vi "Split string by delimiter.vi"(7 "Delimiter":string, 8 "error in (no error)":errorcluster, 10 "String In":string) -> (0 "error out":errorcluster, 2 "String Array Out":string[](array[string]))   [LabVIEW 2015, in "Case Manipulation.lvlib"]
uses:
  Case Manipulation.lvlib
  <vilib>/Utility/error.llb/Error Cluster From Error Code.vi
  <vilib>/ErrorRing/Error Ring.xnode
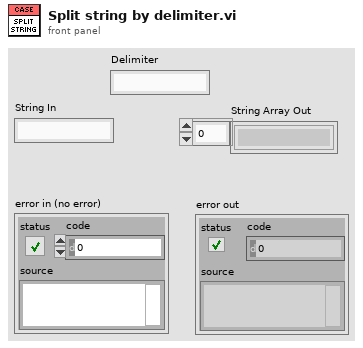
[diagram p1: front panel]
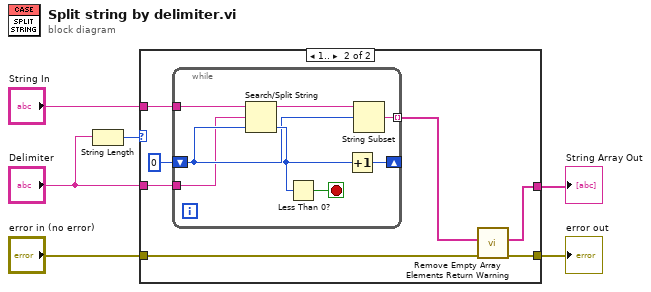
[diagram p0: block diagram]
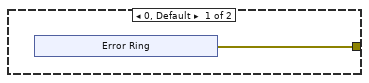
[diagram p2: hidden frame]
diagram:
  n1 = String Length(string="Delimiter") -> (length=w1:i32)
  n2 = case shown="1.." w1 {
    tunnel: "error in (no error)" -> [_ w19]
    tunnel: [w7 w18] -> w5
    tunnel: [_ w17] -> w4
    tunnel: "Delimiter" -> [_ w15]
    tunnel: "String In" -> [_ w13]
    frame 0, Default {
      n3 = xnode "Error Ring"() -> ("error out"=w7:errorcluster)
    }
    frame 1.. {
      n4 = while {
        tunnel: w13 -> [w27]
        shift-right: [w20] -> _
        shift-left: 0 ("offset past match") -> [w24]
        tunnel: [w22] -> w14 mode=indexing
        tunnel: w15 -> [w21]
        stop <- w26 stop-if-true
        n5 = Search/Split String(string=w27, search string/char (-)=w21, offset (0)=w24) -> (substring before match=w23:string, offset of match=w25:i32)  [unwired: 1 out]
        n6 = Less Than 0?(x=w25) -> (x < 0?=w26:bool)
        n7 = Increment(x=w25) -> (x+1=w20:i32)
        n8 = String Subset(string=w23, offset (0)=w24) -> (substring=w22:string)  [unwired: 1 in]
      }
      n9 = call "Remove Empty Array Elements Return Warning.vi"("error in (no error)"=w19, "String Array In"=w14) -> ("error out"=w18:errorcluster, "String Array Out"=w17:string[])  [unwired: 8 in]
    }
  }
  "String Array Out" <- w4
  "error out" <- w5
